vi "GetV.vi"(8 "error in (no error)":errorcluster, 11 "axopatch-200B in":refnum<class "axopatch-200B.lvclass">) -> (0 "error out":errorcluster, 3 "test":dbl)   [LabVIEW 2014, in "axopatch-200B.lvclass"]
uses:
  axopatch-200B.lvclass
  axopatch-200B.lvclass/axopatch-200B.ctl
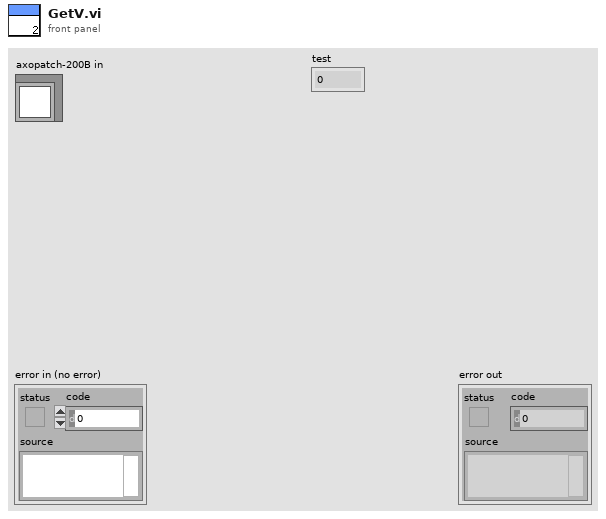
[diagram p1: front panel]
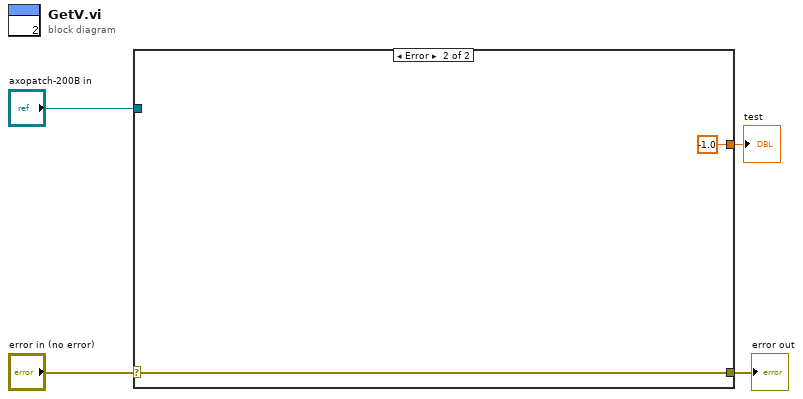
[diagram p0: block diagram]
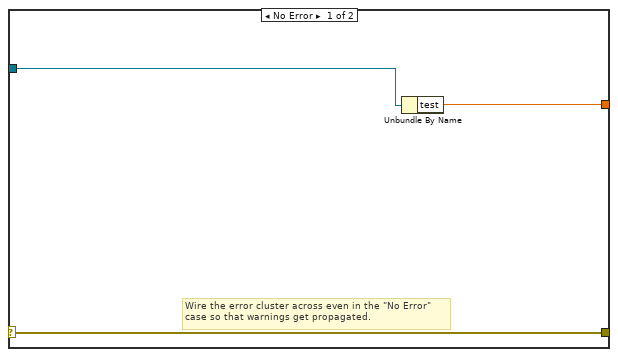
[diagram p2: hidden frame]
diagram:
  n1 = case shown="Error" "error in (no error)" {
    selector: "error in (no error)" -> [w7 w9]
    tunnel: [w7 w9] -> w3
    tunnel: "axopatch-200B in" -> [w6 _]
    tunnel: [w5 -1.0 ("test")] -> w1
    frame No Error {
      # "Wire the error cluster across even in the \"No Error\"\ncase so that warnings get propagated."
      n2 = Unbundle By Name(w6) -> ("test"=w5:dbl)
    }
    frame Error {
    }
  }
  "error out" <- w3
  "test" <- w1
